vi "CurrentEnableDisableTriple.vi"(8 "error in (no error)":errorcluster, 10 "Enable Output (T: On)":bool=TRUE, 11 "Visa Resource Name In":refnum<visa-resource-name>) -> (0 "error in (no error) 2":errorcluster, 3 "Visa Resource Name Out":refnum<visa-resource-name>)   [LabVIEW 2012]
uses:
  Keithley KE22xx Series.lvlib
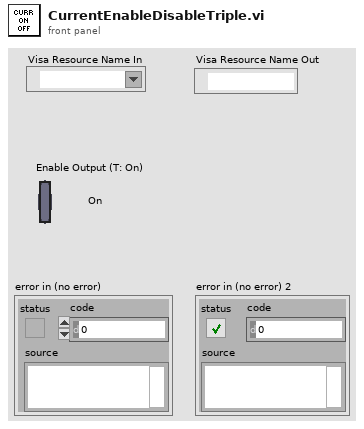
[diagram p1: front panel]
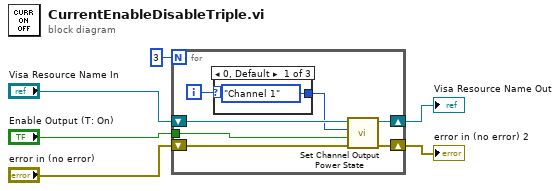
[diagram p0: block diagram]
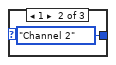
[diagram p2: hidden frame]
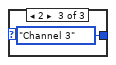
[diagram p3: hidden frame]
diagram:
  n1 = for {
    N: 3 -> [_]
    tunnel: "Enable Output (T: On)" -> [w13]
    shift-right: [w10] -> w2
    shift-left: "error in (no error)" -> [w12]
    shift-right: [w9] -> w1
    shift-left: "Visa Resource Name In" -> [w11]
    i -> [w8]
    n2 = case shown="0, Default" w8 {
      tunnel: [enum16{"Channel 1", "Channel 2", "Channel 3"}."Channel 1" ("Channel Select") enum16{"Channel 1", "Channel 2", "Channel 3"}."Channel 2" ("Channel Select") enum16{"Channel 1", "Channel 2", "Channel 3"}."Channel 3" ("Channel Select")] -> w7
      frame 0, Default {
      }
      frame 1 {
      }
      frame 2 {
      }
    }
    n3 = call "Set Channel Output Power State.vi"("error in (no error)"=w12, "Enable Output (T: On)"=w13, "Channel Select"=w7, "Visa Resource Name IN"=w11) -> ("error out"=w10:errorcluster, "Visa Resource Name OUT"=w9:refnum<visa-resource-name>)  [unwired: 6 in]
  }
  "error in (no error) 2" <- w2
  "Visa Resource Name Out" <- w1
